vi "Read OccupancyGrid.vi"(8 "error in (no error)":errorcluster, 11 "Probabilistic_OccupancyGrid in":refnum<class "Probabilistic_OccupancyGrid.lvclass">) -> (0 "error out":errorcluster, 2 "OccupancyGrid":dbl[][](array[numeric]), 3 "Probabilistic_OccupancyGrid out":refnum<class "Probabilistic_OccupancyGrid.lvclass">)   [LabVIEW 2017, in "Probabilistic_OccupancyGrid.lvclass"]
doc: "Read all values in Occupancy grid\nCell costs are between 0 and 1"
uses:
  Probabilistic_OccupancyGrid.lvclass
  Probabilistic_OccupancyGrid.lvclass/Probabilistic_OccupancyGrid.ctl
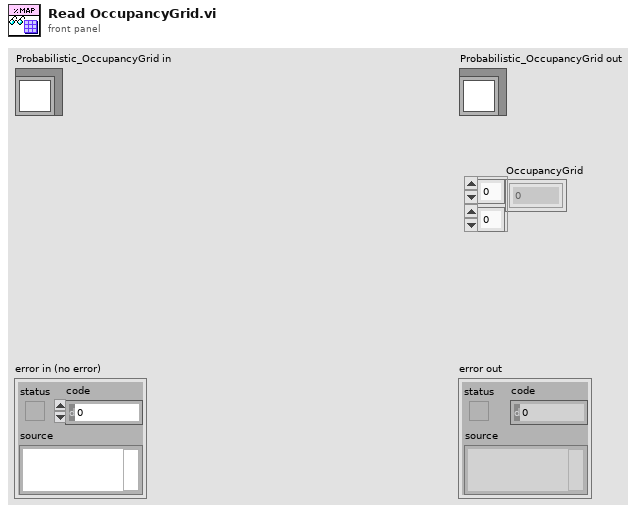
[diagram p1: front panel]
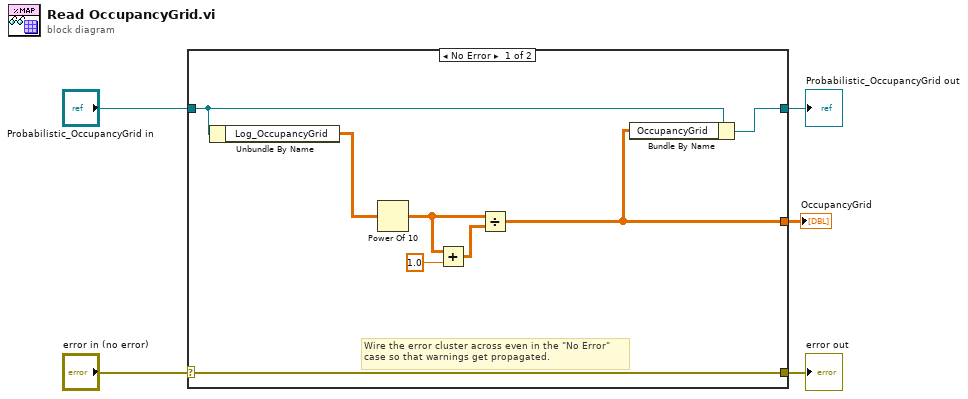
[diagram p0: block diagram]
diagram:
  n1 = case shown="No Error" "error in (no error)" {
    selector: "error in (no error)" -> [w13 w15]
    tunnel: [w13 w15] -> w4
    tunnel: [w7 w14] -> w2
    tunnel: "Probabilistic_OccupancyGrid in" -> [w8 w14]
    tunnel: [w6 _] -> w1
    frame No Error {
      # "Wire the error cluster across even in the \"No Error\"\ncase so that warnings get propagated."
      n2 = Unbundle By Name(w8) -> ("Log_OccupancyGrid"=w12:dbl[][])
      n3 = Power Of 10(x=w12) -> (10^x=w9:dbl[][])
      n4 = Add(x=w9, y=1.0) -> (x+y=w11:dbl[][])
      n5 = Divide(x=w9, y=w11) -> (x/y=w6:dbl[][])
      n6 = Bundle By Name(cluster=w8, "OccupancyGrid"=w6) -> (w7:refnum<class "Probabilistic_OccupancyGrid.lvclass">)
    }
    frame Error {
    }
  }
  "error out" <- w4
  "Probabilistic_OccupancyGrid out" <- w2
  "OccupancyGrid" <- w1
